vi "Configure Source.vi"   [LabVIEW 2017, in "Keithley 2600 Series.lvlib"]
doc: "Configures the basic settings of the source output."
uses:
  <instrlib>/Keithley 2600 Series/Keithley 2600 Series.lvlib
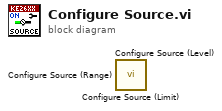
[diagram p0: block diagram]
diagram:
  n1 = call <instrlib>:"Configure Source (Limit).vi"() -> ()  [unwired: 14 in, 2 out]
  n2 = call <instrlib>:"Configure Source (Level).vi"() -> ()  [unwired: 14 in, 2 out]
  n3 = call <instrlib>:"Configure Source (Range).vi"() -> ()  [unwired: 14 in, 2 out]
